vi "OAT Align Range and Current Position.vi"(7 "reset":bool, 9 "range":cluster{"start":dbl, "end":dbl, "step":dbl} {"step" format="%.2f"; "end" format="%.2f"; "start" format="%.2f"}, 11 "current position":dbl format="%.2f") -> (0 "range empty?":bool, 1 "new range":cluster{"start":dbl, "end":dbl, "step":dbl} {"step" format="%.2f"; "end" format="%.2f"; "start" format="%.2f"}, 3 "position out":dbl format="%.2f")   [LabVIEW 2017]
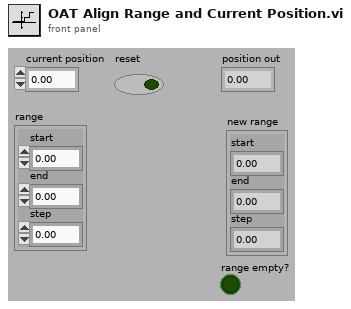
[diagram p1: front panel]
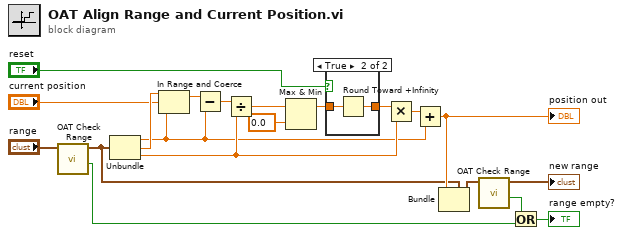
[diagram p0: block diagram]
diagram:
  n1 = call <vilib>:"OAT Check Range.vi"("range in"="range") -> ("empty?"=w15:bool, "range out"=w16:cluster{"start":dbl, "end":dbl, "step":dbl})  [unwired: 8 in, 1 out]
  n2 = Unbundle(w16) -> ("start"=w12:dbl, "end"=w13:dbl, "step"=w17:dbl)
  n3 = In Range and Coerce(upper limit=w13, x="current position", lower limit=w12) -> (coerced(x)=w11:dbl)  [unwired: 1 out]
  n4 = Subtract(x=w11, y=w12) -> (x-y=w8:dbl)
  n5 = Divide(x=w8, y=w17) -> (x/y=w3:dbl)
  n6 = Max & Min(x=w3, y=0.0) -> (max(x,y)=w6:dbl)  [unwired: 1 out]
  n7 = case shown="True" "reset" {
    tunnel: w6 -> [w21 w23]
    tunnel: [w21 w22] -> w2
    frame False {
    }
    frame True {
      n8 = Round Toward +Infinity(x=w23) -> (ceil(x): smallest int >= x=w22:dbl)
    }
  }
  n9 = Multiply(x=w2, y=w17) -> (x*y=w5:dbl)
  n10 = Add(x=w5, y=w12) -> (x+y=w20:dbl)
  "position out" <- w20
  n11 = Bundle(cluster=w16, "start"=w20) -> (w4:cluster{"start":dbl, "end":dbl, "step":dbl})  [unwired: 2 in]
  n12 = call <vilib>:"OAT Check Range.vi"("range in"=w4) -> ("empty?"=w9:bool, "range out"=→"new range":cluster{"start":dbl, "end":dbl, "step":dbl})  [unwired: 8 in, 1 out]
  n13 = Or(x=w9, y=w15) -> (x .or. y?=→"range empty?":bool)
